vi "Test Lockin Digitizer Driver.vi"() -> ()   [LabVIEW 2021]
uses:
  Instruments/Pulse Driver/Lockin Digitizer Driver/Lockin Digitizer Configuration.ctl
  LabActor/Worker/Worker Actor/Background Loop Action.ctl
  DAQmx Lockin Digitizer Driver/DAQmx Lockin Digitizer Driver.lvclass
  C:/GitHub/NHMFL_Core/Libraries/Instruments/Instrument Driver/Instrument Driver.lvclass
  C:/GitHub/NHMFL_Core/Libraries/NI-DAQ/DAQmx Digitizer/DAQmx Digitizer.lvclass
  C:/GitHub/NHMFL_Core/Libraries/Instruments/Pulse Driver/Lockin Digitizer Driver/Lockin Digitizer Driver.lvclass
  DAQmx Digitizer/DAQmx Digitizer.lvclass/DAQmx Digitizer.ctl
  DAQmx Digitizer/Write DAQmx Device Name.vi
  <resource>/objmgr/daqmx.rc
panel:
  out "AO task":refnum<k21>
  out "ChannelsToRead":refnum<k21>
  in  "Stop Button":bool
  in  "DAQmx Device Name":tag
  out "Y":dbl[](array[numeric]) format="%#_6pV"
  out "X":dbl[](array[numeric]) format="%#_6pV"
  out "Action out":T1
  in  "Period":i32
  in  "Configuration":T2={"Post-trigger delay"=0.01, "Post-trigger duration"=0.1, "Rate"=1000000.0, "Ranges"=[10.0], "Re-name channels"=[], "Active channels"="0:1", "External\nclock"=FALSE, "Frequencies"=[100000.0], "Monitor time\nconstant"=1.0, "Output \namplitudes"=[1.0], "Input\nchannles"=["0"], "Sync"=FALSE, "Lock-in input channel phases"=[]} {"Output \namplitudes" format="%#_6pV"; "Monitor time\nconstant" format="%#_6ps"; "Frequencies" format="%#_6pHz"; "Rate" format="%#_8pHz"; "Post-trigger duration" format="%#_6ps"; "Post-trigger delay" format="%#_6ps"; "Ranges" format="%#_6pV"}
  # "Pulse config"
  # "Lock-in config"
  # "#0\n\n#1"
  # "Monitor config"
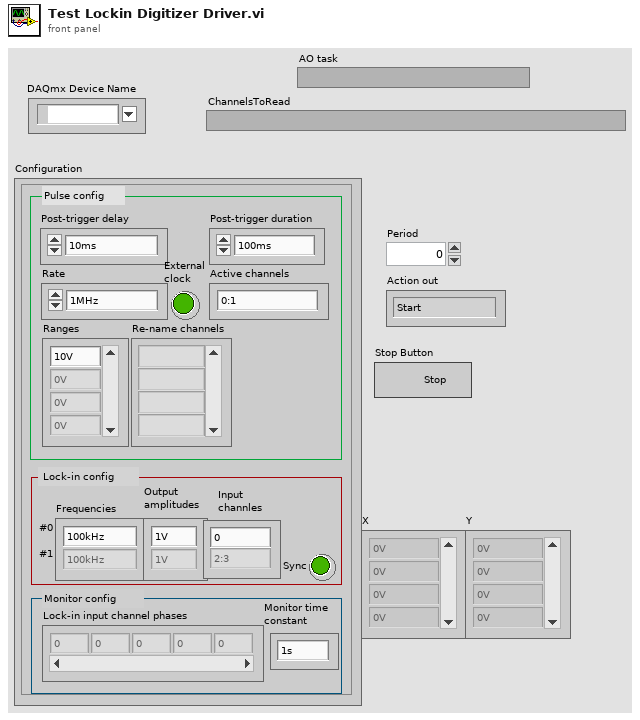
[diagram p1: front panel]
types:
  T1 = typedef "Background Loop Action.ctl" = enum16{"Start", "Continue", "Stop"}
  T2 = typedef "Lockin Digitizer Configuration.ctl" = cluster{"Post-trigger delay":dbl, "Post-trigger duration":dbl, "Rate":dbl, "Ranges":dbl[], "Re-name channels":string[], "Active channels":string, "External\nclock":bool, "Frequencies":dbl[], "Monitor time\nconstant":dbl, "Output \namplitudes":dbl[], "Input\nchannles":string[], "Sync":bool, "Lock-in input channel phases":dbl[]}
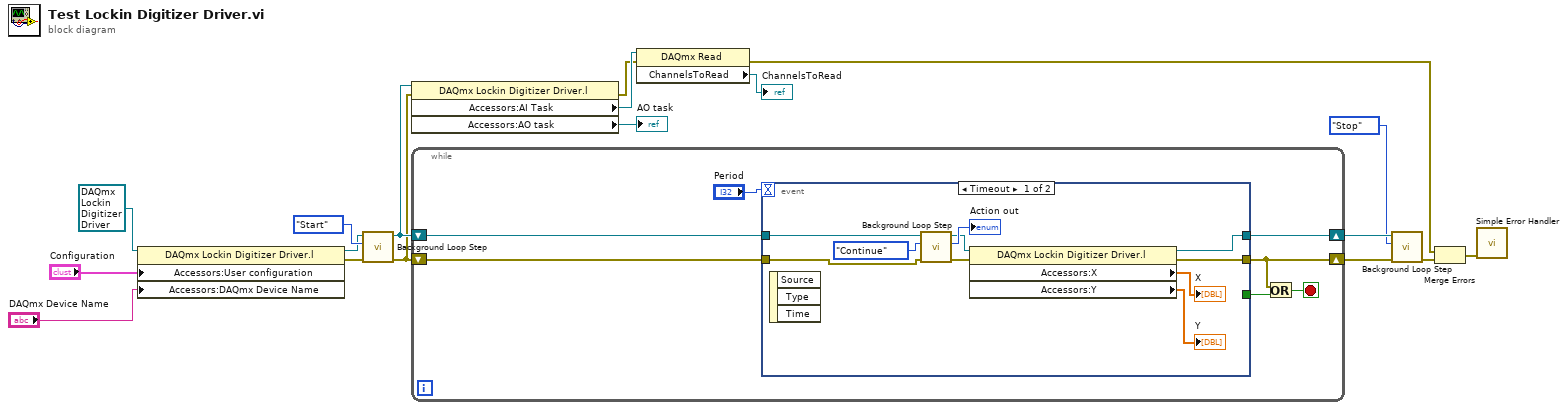
[diagram p0: block diagram]
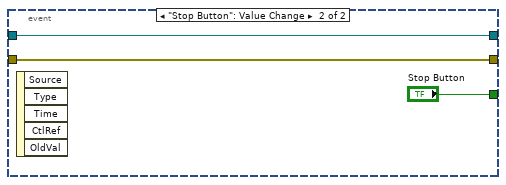
[diagram p2: hidden frame]
diagram:
  n1 = property class="DAQmx Lockin Digitizer Driver.l"(reference=refnum<class "DAQmx Lockin Digitizer Driver.lvclass"> refnum ("DAQmx Lockin Digitizer Driver.lvclass"), "Accessors:User configuration"="Configuration", "Accessors:DAQmx Device Name"="DAQmx Device Name") -> (reference out=w14:refnum<class "DAQmx Lockin Digitizer Driver.lvclass">, error out=w13:errorcluster)  [unwired: 1 in]
  n2 = call-dynamic "Background Loop Step.vi"("error in (no error)"=w13, "Action"=Background_Loop_Action."Start", "DAQmx Lockin Digitizer Driver in"=w14) -> ("error out"=w5:errorcluster, "DAQmx Lockin Digitizer Driver out"=w8:refnum<class "DAQmx Lockin Digitizer Driver.lvclass">)  [unwired: 4 in, 3 out]
  n3 = property class="DAQmx Lockin Digitizer Driver.l"(reference=w8, error in=w5) -> (error out=w6:errorcluster, "Accessors:AI Task"=w7:refnum<k21>, "Accessors:AO task"=→"AO task":refnum<k21>)  [unwired: 1 out]
  n4 = while {
    shift-right: [w22] -> w12
    shift-left: w8 -> [w23]
    shift-right: [w20] -> w11
    shift-left: w5 -> [w24]
    stop <- w21 stop-if-true
    n5 = event shown="[0] Timeout" {
      selector: _ -> [_ _]
      dyn-events: _ -> [_ _]
      timeout: "Period" -> [_ _]
      tunnel: w24 -> [w35 w37]
      tunnel: w23 -> [w34 w36]
      tunnel: [w30 w37] -> w20
      tunnel: [w28 w36] -> w22
      tunnel: [_ "Stop Button"] -> w19
      event Timeout {
        n6 = event-data() -> ()  [unwired: 1 in, 3 out]
        n7 = call-dynamic "Background Loop Step.vi"("error in (no error)"=w35, "Action"=Background_Loop_Action."Continue", "DAQmx Lockin Digitizer Driver in"=w34) -> ("error out"=w33:errorcluster, "Action out"=→"Action out":T1, "DAQmx Lockin Digitizer Driver out"=w29:refnum<class "DAQmx Lockin Digitizer Driver.lvclass">)  [unwired: 4 in, 2 out]
        n8 = property class="DAQmx Lockin Digitizer Driver.l"(reference=w29, error in=w33) -> (reference out=w28:refnum<class "DAQmx Lockin Digitizer Driver.lvclass">, error out=w30:errorcluster, "Accessors:X"=→"X":dbl[], "Accessors:Y"=→"Y":dbl[])
      }
      event "Stop Button": Value Change {
        n9 = event-data() -> ()  [unwired: 1 in, 5 out]
      }
    }
    n10 = Or(x=w20, y=w19) -> (x .or. y?=w21:bool)
  }
  n11 = property class="DAQmx Read"(reference=w7, error in=w6) -> (error out=w3:errorcluster, "ChannelsToRead"=→"ChannelsToRead":refnum<k21>)  [unwired: 1 out]
  n12 = call-dynamic "Background Loop Step.vi"("error in (no error)"=w11, "Action"=Background_Loop_Action."Stop", "DAQmx Lockin Digitizer Driver in"=w12) -> ("error out"=w9:errorcluster)  [unwired: 4 in, 4 out]
  n13 = Merge Errors(w3, w9) -> (w4:errorcluster)
  n14 = call <vilib>:"Simple Error Handler.vi"("error in (no error)"=w4) -> ()  [unwired: 4 in, 5 out]
